vi "Write PV to OPCUA-Server.vi"(8 "Error In":errorcluster, 10 "PV":refnum<class "PV.lvclass">, 11 "CS++OPCUAInterface in":refnum<class "CS++OPCUAInterface.lvclass">) -> (0 "Error Out":errorcluster, 3 "CS++OPCUAInterface out":refnum<class "CS++OPCUAInterface.lvclass">)   [LabVIEW 2015, in "CS++OPCUAInterface.lvlib" / "CS++OPCUAInterface.lvclass"]
doc: "Write the PV to the OPC-UA server."
uses:
  CS++OPCUAInterface.lvclass
  CSPP_Core/Classes/CS++ProcessVariables/ProcessVariable/PV.lvclass
  CS++OPCUAInterface.lvclass/CS++OPCUAInterface.ctl
  CSPP_Core/Classes/CS++ProcessVariables/ProcessVariable/PV.lvclass/PV.ctl
  CSPP_Core/Actors/CS++BaseActor/CS++BaseActor.lvclass/CS++BaseActor.ctl
  CSPP_Core/Classes/CS++ProcessVariables/ProcessVariable/Read PV URL.vi
  CSPP_Core/Classes/CS++ProcessVariables/ProcessVariable/Read Data.vi
  CSPP_Core/Classes/CS++ProcessVariables/ProcessVariable/Read Type Descriptor.vi
  <vilib>/OPCUA/client/Write Bool.vi
  <vilib>/OPCUA/client/Write Byte.vi
  <vilib>/OPCUA/client/Write SByte.vi
  <vilib>/OPCUA/client/Write Int16.vi
  <vilib>/OPCUA/client/Write UInt16.vi
  <vilib>/OPCUA/client/Write Int32.vi
  <vilib>/OPCUA/client/Write UInt32.vi
  <vilib>/OPCUA/client/Write Int64.vi
  <vilib>/OPCUA/client/Write UInt64.vi
  <vilib>/OPCUA/client/Write Float.vi
  <vilib>/OPCUA/client/Write Double.vi
  <vilib>/OPCUA/client/Write Bool Array.vi
  <vilib>/OPCUA/client/Write Byte Array.vi
  <vilib>/OPCUA/client/Write Int16 Array.vi
  <vilib>/OPCUA/client/Write Int32 Array.vi
  <vilib>/OPCUA/client/Write Int64 Array.vi
  <vilib>/OPCUA/client/Write Float Array.vi
  <vilib>/OPCUA/client/Write Double Array.vi
  <vilib>/OPCUA/NI OPC UA Client.lvlib
  CSPP_Core/Libraries/Utilities/CS++Utilities.lvlib
  CSPP_Core/Actors/CS++BaseActor/CS++BaseActor.lvclass
panel:
  out "Timing Chart":dbl[unit](graph)
  out "dt":dbl[unit] format="%.3p"
  out "current time":timestamp format="%<%I:%M:%S%3u %p\n%m/%d/%Y>T"
  out "Accessors:Data":variant
  out "OPC Item":string
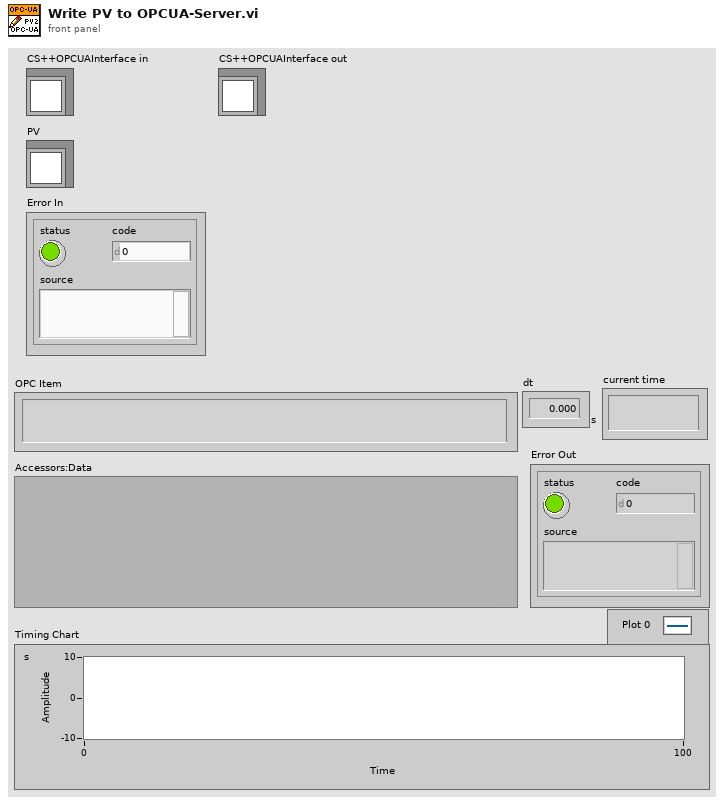
[diagram p1: front panel]
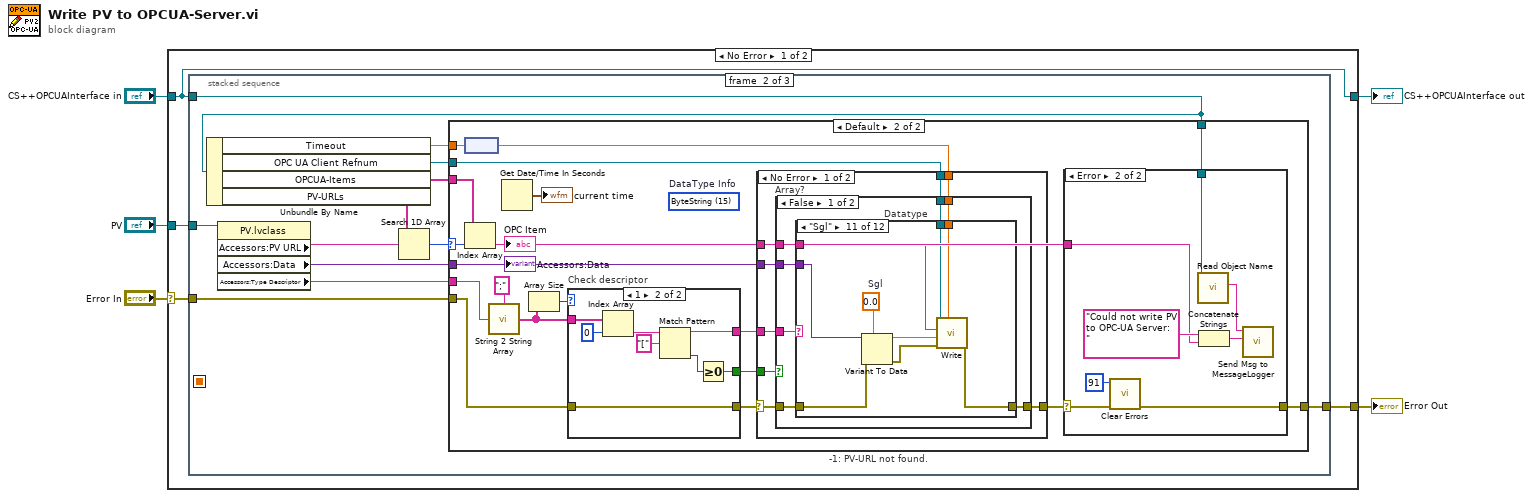
[diagram p0: block diagram]
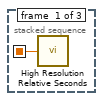
[diagram p2: hidden frame]
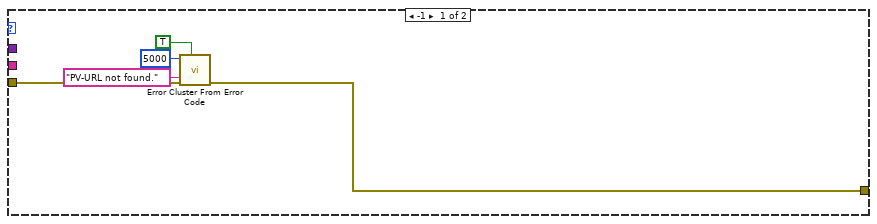
[diagram p3: hidden frame]
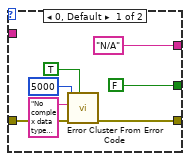
[diagram p5: hidden frame]
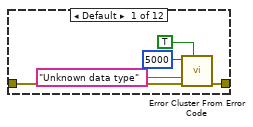
[diagram p6: hidden frame]
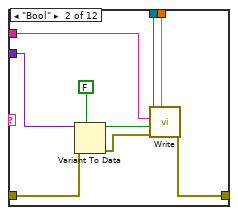
[diagram p7: hidden frame]
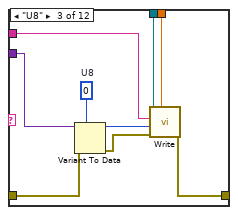
[diagram p8: hidden frame]
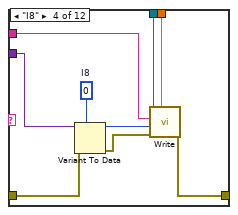
[diagram p9: hidden frame]
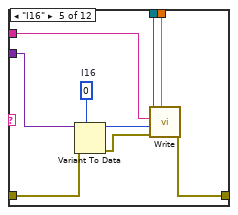
[diagram p10: hidden frame]
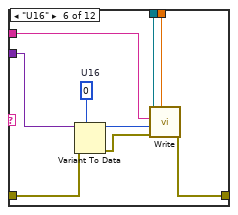
[diagram p11: hidden frame]
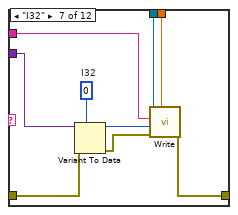
[diagram p12: hidden frame]
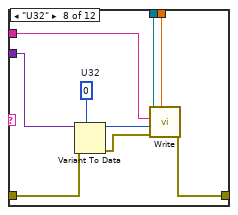
[diagram p13: hidden frame]
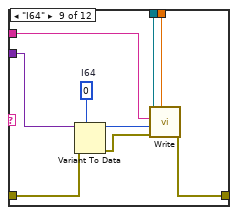
[diagram p14: hidden frame]
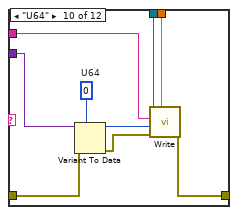
[diagram p15: hidden frame]
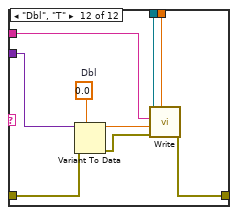
[diagram p16: hidden frame]
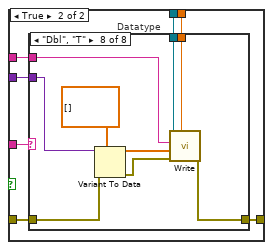
[diagram p17: hidden frame]
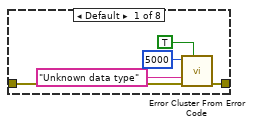
[diagram p18: hidden frame]
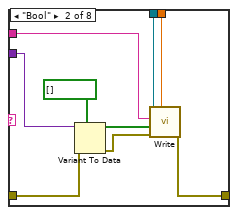
[diagram p19: hidden frame]
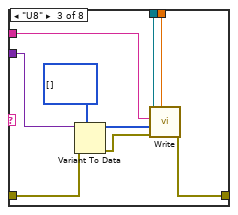
[diagram p20: hidden frame]
diagram:
  n1 = case shown="No Error" "Error In" {
    selector: "Error In" -> [w7 w271]
    tunnel: [w9 w271] -> w4
    tunnel: [w6 w270] -> w2
    tunnel: "CS++OPCUAInterface in" -> [w6 w270]
    tunnel: "PV" -> [w8 _]
    frame No Error {
      n2 = stacked-sequence {
        seq-local: [w10 _ _] -> [_ _ w268]
        tunnel: [_ w21 _] -> w9
        tunnel: w8 -> [_ w20 _]
        tunnel: w7 -> [_ w14 _]
        tunnel: w6 -> [_ w11 _]
        frame #0 {
          n3 = call <vilib>:"High Resolution Relative Seconds.vi"() -> ("relative seconds"=w10:dbl)
        }
        frame #1 {
          n4 = Unbundle By Name(w11) -> ("Timeout"=w15:dbl[unit], "OPC UA Client Refnum"=w22:refnum<k21>, "OPCUA-Items"=w17:string[], "PV-URLs"=w19:string[])
          n5 = property class="PV.lvclass"(reference=w20) -> ("Accessors:PV URL"=w18:string, "Accessors:Data"=w16:variant, "Accessors:Type Descriptor"=w13:string)  [unwired: 1 in, 2 out]
          n6 = Search 1D Array(1D array=w19, element=w18) -> (index of element=w12:i32)  [unwired: 1 in]
          n7 = case "-1: PV-URL not found." shown="Default" w12 {
            selector: w12 -> [_ w41]
            tunnel: w22 -> [_ w46]
            tunnel: [w26 w32] -> w21
            tunnel: w17 -> [_ w45]
            tunnel: w16 -> [_ w44]
            tunnel: w15 -> [_ w43]
            tunnel: w14 -> [w27 w36]
            tunnel: w13 -> [_ w33]
            tunnel: w11 -> [_ w30]
            frame -1 {
              n8 = call <vilib>:"Error Cluster From Error Code.vi"("show call chain? (False)"=TRUE, "error in (no error)"=w27, "error message (\"\")"="PV-URL not found." ("error message (\"\")"), "error code (0)"=5000) -> ("error out"=w26:errorcluster)  [unwired: 5 in]
            }
            frame Default {
              (unwired) u32 15 items=["Boolean"=1, "SByte"=2, "Byte"=3, "Int16"=4, "UInt16"=5, "Int32"=6, "UInt32"=7, "Int64"=8, "UInt64"=9, "Float"=10, "Double"=11, "String"=12, "DateTime"=13, "ByteString"=15, "Array of Boolean"=101, "Array of SByte"=102, "Array of Byte"=103, "Array of Int16"=104, "Array of UInt16"=105, "Array of Int32"=106, "Array of UInt32"=107, "Array of Int64"=108, "Array of UInt64"=109, "Array of Float"=110, "Array of Double"=111, "Array of String"=112, "Array of DateTime"=113, "Array of ByteString"=115]  # DataType Info
              n9 = node(w43) -> (w42:dbl)
              n10 = Index Array(array=w45, index=w41) -> (element=w29:string)
              "OPC Item" <- w29
              n11 = call "String 2 String Array.vi"("String"=w33, "Delimiter (\",\")"=";" ("Delimiter (\",\")")) -> ("Substrings"=w38:string[])
              n12 = Get Date/Time In Seconds() -> (seconds since 1Jan1904=→"current time":timestamp)
              n13 = Array Size(array=w38) -> (size(s)=w40:i32)
              n14 = case "Check descriptor" shown="1" w40 {
                tunnel: w36 -> [w62 w70]
                tunnel: [w61 w70] -> w35
                tunnel: w38 -> [_ w68]
                tunnel: ["N/A" ("Substring") w63] -> w37
                tunnel: [FALSE w65] -> w34
                frame 0, Default {
                  n15 = call <vilib>:"Error Cluster From Error Code.vi"("show call chain? (False)"=TRUE, "error in (no error)"=w62, "error message (\"\")"="No complex data types support for now." ("error message (\"\")"), "error code (0)"=5000) -> ("error out"=w61:errorcluster)  [unwired: 5 in]
                }
                frame 1 {
                  n16 = Index Array(array=w68, index=0) -> (element=w66:string)
                  n17 = Match Pattern(string=w66, regular expression="[") -> (before substring=w63:string, offset past match=w64:i32)  [unwired: 1 in, 2 out]
                  n18 = Greater Or Equal To 0?(x=w64) -> (x >= 0?=w65:bool)
                }
              }
              n19 = case shown="No Error" w35 {
                selector: w35 -> [w72 w265]
                tunnel: w46 -> [w78 _]
                tunnel: [w77 w265] -> w31
                tunnel: w29 -> [w76 _]
                tunnel: w44 -> [w75 _]
                tunnel: w42 -> [w74 _]
                tunnel: w37 -> [w73 _]
                tunnel: w34 -> [w71 _]
                frame No Error {
                  n20 = case "Array?" shown="False" w71 {
                    tunnel: w78 -> [w85 w196]
                    tunnel: [w84 w195] -> w77
                    tunnel: w76 -> [w83 w194]
                    tunnel: w75 -> [w82 w193]
                    tunnel: w74 -> [w81 w192]
                    tunnel: w73 -> [w80 w191]
                    tunnel: w72 -> [w79 w190]
                    frame False {
                      n21 = case "Datatype" shown="\"Sgl\"" w80 {
                        tunnel: w85 -> [_ w99 w108 w117 w126 w135 w144 w153 w162 w171 w180 w189]
                        tunnel: [w89 w98 w107 w116 w125 w134 w143 w152 w161 w170 w179 w188] -> w84
                        tunnel: w83 -> [_ w97 w106 w115 w124 w133 w142 w151 w160 w169 w178 w187]
                        tunnel: w82 -> [_ w96 w105 w114 w123 w132 w141 w150 w159 w168 w177 w186]
                        tunnel: w81 -> [_ w93 w103 w112 w121 w130 w139 w148 w157 w166 w175 w184]
                        tunnel: w79 -> [w90 w92 w102 w111 w120 w129 w138 w147 w156 w165 w174 w183]
                        frame Default {
                          n22 = call <vilib>:"Error Cluster From Error Code.vi"("show call chain? (False)"=TRUE, "error in (no error)"=w90, "error message (\"\")"="Unknown data type" ("error message (\"\")"), "error code (0)"=5000) -> ("error out"=w89:errorcluster)  [unwired: 5 in]
                        }
                        frame "Bool" {
                          n23 = Variant To Data(error in=w92, type=FALSE, Variant=w96) -> (data=w94:bool, error out=w91:errorcluster)
                          n24 = call-poly <vilib>:"Write.vi"("timeout (5000 ms)"=w93, "error in (no error)"=w91, "value"=w94, "node path"=w97, "OPC UA client refnum in"=w99) -> ("error out"=w98:errorcluster)  [unwired: 4 in, 2 out]
                        }
                        frame "U8" {
                          w100 = u8 0  # U8
                          n25 = Variant To Data(error in=w102, type=w100, Variant=w105) -> (data=w104:u8, error out=w101:errorcluster)
                          n26 = call-poly <vilib>:"Write.vi"("timeout (5000 ms)"=w103, "error in (no error)"=w101, "value"=w104, "node path"=w106, "OPC UA client refnum in"=w108) -> ("error out"=w107:errorcluster)  [unwired: 4 in, 2 out]
                        }
                        frame "I8" {
                          w109 = i8 0  # I8
                          n27 = Variant To Data(error in=w111, type=w109, Variant=w114) -> (data=w113:i8, error out=w110:errorcluster)
                          n28 = call-poly <vilib>:"Write.vi"("timeout (5000 ms)"=w112, "error in (no error)"=w110, "value"=w113, "node path"=w115, "OPC UA client refnum in"=w117) -> ("error out"=w116:errorcluster)  [unwired: 4 in, 2 out]
                        }
                        frame "I16" {
                          w118 = i16 0  # I16
                          n29 = Variant To Data(error in=w120, type=w118, Variant=w123) -> (data=w122:i16, error out=w119:errorcluster)
                          n30 = call-poly <vilib>:"Write.vi"("timeout (5000 ms)"=w121, "error in (no error)"=w119, "value"=w122, "node path"=w124, "OPC UA client refnum in"=w126) -> ("error out"=w125:errorcluster)  [unwired: 4 in, 2 out]
                        }
                        frame "U16" {
                          w127 = u16 0  # U16
                          n31 = Variant To Data(error in=w129, type=w127, Variant=w132) -> (data=w131:u16, error out=w128:errorcluster)
                          n32 = call-poly <vilib>:"Write.vi"("timeout (5000 ms)"=w130, "error in (no error)"=w128, "value"=w131, "node path"=w133, "OPC UA client refnum in"=w135) -> ("error out"=w134:errorcluster)  [unwired: 4 in, 2 out]
                        }
                        frame "I32" {
                          w136 = 0  # I32
                          n33 = Variant To Data(error in=w138, type=w136, Variant=w141) -> (data=w140:i32, error out=w137:errorcluster)
                          n34 = call-poly <vilib>:"Write.vi"("timeout (5000 ms)"=w139, "error in (no error)"=w137, "value"=w140, "node path"=w142, "OPC UA client refnum in"=w144) -> ("error out"=w143:errorcluster)  [unwired: 4 in, 2 out]
                        }
                        frame "U32" {
                          w145 = u32 0  # U32
                          n35 = Variant To Data(error in=w147, type=w145, Variant=w150) -> (data=w149:u32, error out=w146:errorcluster)
                          n36 = call-poly <vilib>:"Write.vi"("timeout (5000 ms)"=w148, "error in (no error)"=w146, "value"=w149, "node path"=w151, "OPC UA client refnum in"=w153) -> ("error out"=w152:errorcluster)  [unwired: 4 in, 2 out]
                        }
                        frame "I64" {
                          w154 = 0  # I64
                          n37 = Variant To Data(error in=w156, type=w154, Variant=w159) -> (data=w158:i32, error out=w155:errorcluster)
                          n38 = call-poly <vilib>:"Write.vi"("timeout (5000 ms)"=w157, "error in (no error)"=w155, "value"=w158, "node path"=w160, "OPC UA client refnum in"=w162) -> ("error out"=w161:errorcluster)  [unwired: 4 in, 2 out]
                        }
                        frame "U64" {
                          w163 = u64 0  # U64
                          n39 = Variant To Data(error in=w165, type=w163, Variant=w168) -> (data=w167:u64, error out=w164:errorcluster)
                          n40 = call-poly <vilib>:"Write.vi"("timeout (5000 ms)"=w166, "error in (no error)"=w164, "value"=w167, "node path"=w169, "OPC UA client refnum in"=w171) -> ("error out"=w170:errorcluster)  [unwired: 4 in, 2 out]
                        }
                        frame "Sgl" {
                          w172 = sgl 0.0  # Sgl
                          n41 = Variant To Data(error in=w174, type=w172, Variant=w177) -> (data=w176:sgl, error out=w173:errorcluster)
                          n42 = call-poly <vilib>:"Write.vi"("timeout (5000 ms)"=w175, "error in (no error)"=w173, "value"=w176, "node path"=w178, "OPC UA client refnum in"=w180) -> ("error out"=w179:errorcluster)  [unwired: 4 in, 2 out]
                        }
                        frame "Dbl", "T" {
                          w181 = 0.0  # Dbl
                          n43 = Variant To Data(error in=w183, type=w181, Variant=w186) -> (data=w185:dbl, error out=w182:errorcluster)
                          n44 = call-poly <vilib>:"Write.vi"("timeout (5000 ms)"=w184, "error in (no error)"=w182, "value"=w185, "node path"=w187, "OPC UA client refnum in"=w189) -> ("error out"=w188:errorcluster)  [unwired: 4 in, 2 out]
                        }
                      }
                    }
                    frame True {
                      n45 = case "Datatype" shown="\"Dbl\", \"T\"" w191 {
                        tunnel: w196 -> [_ w210 w219 w228 w237 w246 w255 w264]
                        tunnel: [w200 w209 w218 w227 w236 w245 w254 w263] -> w195
                        tunnel: w194 -> [_ w208 w217 w226 w235 w244 w253 w262]
                        tunnel: w193 -> [_ w207 w216 w225 w234 w243 w252 w261]
                        tunnel: w192 -> [_ w205 w214 w223 w232 w241 w250 w259]
                        tunnel: w190 -> [w201 w204 w213 w222 w231 w240 w249 w258]
                        frame Default {
                          n46 = call <vilib>:"Error Cluster From Error Code.vi"("show call chain? (False)"=TRUE, "error in (no error)"=w201, "error message (\"\")"="Unknown data type" ("error message (\"\")"), "error code (0)"=5000) -> ("error out"=w200:errorcluster)  [unwired: 5 in]
                        }
                        frame "Bool" {
                          n47 = Variant To Data(error in=w204, type=bool[] [], Variant=w207) -> (data=w206:bool[], error out=w203:errorcluster)
                          n48 = call-poly <vilib>:"Write.vi"("timeout (5000 ms)"=w205, "error in (no error)"=w203, "value"=w206, "node path"=w208, "OPC UA client refnum in"=w210) -> ("error out"=w209:errorcluster)  [unwired: 4 in, 2 out]
                        }
                        frame "U8" {
                          n49 = Variant To Data(error in=w213, type=u8[] [], Variant=w216) -> (data=w215:u8[], error out=w212:errorcluster)
                          n50 = call-poly <vilib>:"Write.vi"("timeout (5000 ms)"=w214, "error in (no error)"=w212, "value"=w215, "node path"=w217, "OPC UA client refnum in"=w219) -> ("error out"=w218:errorcluster)  [unwired: 4 in, 2 out]
                        }
                        frame "I8" {
                          n51 = Variant To Data(error in=w222, type=i16[] [], Variant=w225) -> (data=w224:i16[], error out=w221:errorcluster)
                          n52 = call-poly <vilib>:"Write.vi"("timeout (5000 ms)"=w223, "error in (no error)"=w221, "value"=w224, "node path"=w226, "OPC UA client refnum in"=w228) -> ("error out"=w227:errorcluster)  [unwired: 4 in, 2 out]
                        }
                        frame "I32" {
                          n53 = Variant To Data(error in=w231, type=i32[] [], Variant=w234) -> (data=w233:i32[], error out=w230:errorcluster)
                          n54 = call-poly <vilib>:"Write.vi"("timeout (5000 ms)"=w232, "error in (no error)"=w230, "value"=w233, "node path"=w235, "OPC UA client refnum in"=w237) -> ("error out"=w236:errorcluster)  [unwired: 4 in, 2 out]
                        }
                        frame "I64" {
                          n55 = Variant To Data(error in=w240, type=i32[] [], Variant=w243) -> (data=w242:i32[], error out=w239:errorcluster)
                          n56 = call-poly <vilib>:"Write.vi"("timeout (5000 ms)"=w241, "error in (no error)"=w239, "value"=w242, "node path"=w244, "OPC UA client refnum in"=w246) -> ("error out"=w245:errorcluster)  [unwired: 4 in, 2 out]
                        }
                        frame "Sgl" {
                          n57 = Variant To Data(error in=w249, type=sgl[] [], Variant=w252) -> (data=w251:sgl[], error out=w248:errorcluster)
                          n58 = call-poly <vilib>:"Write.vi"("timeout (5000 ms)"=w250, "error in (no error)"=w248, "value"=w251, "node path"=w253, "OPC UA client refnum in"=w255) -> ("error out"=w254:errorcluster)  [unwired: 4 in, 2 out]
                        }
                        frame "Dbl", "T" {
                          n59 = Variant To Data(error in=w258, type=dbl[] [], Variant=w261) -> (data=w260:dbl[], error out=w257:errorcluster)
                          n60 = call-poly <vilib>:"Write.vi"("timeout (5000 ms)"=w259, "error in (no error)"=w257, "value"=w260, "node path"=w262, "OPC UA client refnum in"=w264) -> ("error out"=w263:errorcluster)  [unwired: 4 in, 2 out]
                        }
                      }
                    }
                  }
                }
                frame Error {
                }
              }
              n61 = case shown="Error" w31 {
                selector: w31 -> [w47 w53]
                tunnel: [w47 w54] -> w32
                tunnel: w30 -> [_ w50]
                tunnel: w29 -> [_ w48]
                frame No Error {
                }
                frame Error {
                  n62 = call <vilib>:"Clear Errors.vi"("error in (no error)"=w53, "specific error code to clear (0: all)"=91) -> ("error out"=w54:errorcluster)  [unwired: 4 in, 1 out]
                  n63 = call "Read Object Name.vi"("CS++BaseActor in"=w50) -> ("Object Name"=w49:string)  [unwired: 8 in, 2 out]
                  n64 = Concatenate Strings("Could not write PV to OPC-UA Server:  " ("Message Content"), w48) -> (w51:string)
                  n65 = call "Send Msg to MessageLogger.vi"("Message Content"=w51, "Message Tag"=w49) -> ()  [unwired: 9 in, 1 out]
                }
              }
              "Accessors:Data" <- w44
            }
          }
        }
        frame #2 {
          n66 = call <vilib>:"High Resolution Relative Seconds.vi"() -> ("relative seconds"=w269:dbl)
          n67 = Subtract(x=w269, y=w268) -> (x-y=w267:dbl)
          n68 = node(w267) -> (→"dt" →"Timing Chart":dbl[unit])
        }
      }
    }
    frame Error {
    }
  }
  "Error Out" <- w4
  "CS++OPCUAInterface out" <- w2
